vi "DFD Filter Array.vi"(7 "init (F)":bool, 8 "error in (no error)":errorcluster, 10 "filters":T1[](array[typedef]) {"mSRate_QSettings"."source" items=["Coef a/k"=0, "Coef b/v"=7, "Input"=1, "Output"=2, "Multiplicand"=3, "Product"=4, "Sum"=5, "Delay"=6, "Gain"=8]}, 11 "signal in":waveform(dbl)[](array[waveform])) -> (0 "error out":errorcluster, 3 "signal out":waveform(dbl)[](array[waveform]))   [LabVIEW 2019, in "Instrument.Lockin.lvlib" / "Instrument.DAQ.lvclass"]
uses:
  Instrument.DAQ.lvclass
  <vilib>/addons/Digital Filter Design/_Objects.llb/DFD Filter Obj.ctl
  <vilib>/addons/Digital Filter Design/_Objects.llb/DFD Filter Coef.ctl
  <vilib>/addons/Digital Filter Design/_Objects.llb/DFD Filter Structure Type Selector.ctl
  <vilib>/addons/Digital Filter Design/_Objects.llb/dfd_Internal Quantization Settings.ctl
  <vilib>/addons/Digital Filter Design/_Objects.llb/dfd_Internal Quantization Srcs.ctl
  <vilib>/addons/Digital Filter Design/_Objects.llb/DFD Coef Norm Type.ctl
  <vilib>/addons/Digital Filter Design/Process.llb/DFD Filtering with State (Wfm).vi
  <vilib>/addons/Digital Filter Design/NI_DigFilterLicensed.lvlib
  <vilib>/addons/Digital Filter Design/NI_DigFilter_Process.lvlib
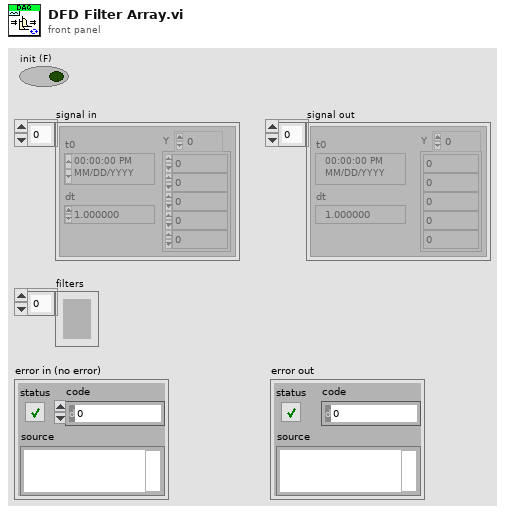
[diagram p1: front panel]
types:
  T1 = typedef "NI_DigFilterLicensed.lvlib/DFD Filter Obj.ctl" = cluster{"mSRate_Fs":dbl, "mSRate_Version":string, "mSRate_Comments":string, "mSRate_OrgCoef":T2, "mSRate_CurCoef":T2, "mSRate_Quantized?":bool, "mSRate_QCoef":T2, "mSRate_QSettings":T4[], "mSRate_Order":i32, "mSRate_Scaling":cluster{"mSRate_ScaleByPowerOf2?":bool, "mSRate_ScaleType":T6}}
  T2 = typedef "NI_DigFilterLicensed.lvlib/DFD Filter Coef.ctl" = cluster{"type":T3, "gain":dbl, "coef a (k)":dbl[], "coef b (v)":dbl[]}
  T3 = typedef "NI_DigFilterLicensed.lvlib/DFD Filter Structure Type Selector.ctl" = enum16{"Undefined", "FIR Direct Form", "FIR Direct Form Transposed", "FIR Symmetric", "FIR Antisymmetric", "IIR Direct Form I", "IIR Direct Form I Transposed", "IIR Direct Form II", "IIR Direct Form II Transposed", "IIR Cascaded Second Order Sections Form I", "IIR Cascaded Second Order Sections Form I Transposed", "IIR Cascaded Second Order Sections Form II", "IIR Cascaded Second Order Sections Form II Transposed", "Lattice Allpass (basic sections)", "Lattice Allpass (one multiplier sections)", "Lattice Allpass (normalized sections)", "Lattice AR (basic sections)", "Lattice AR (one multiplier sections)", "Lattice AR (normalized sections)", "Lattice MA (minimum phase)", "Lattice MA (maximum phase)", "Lattice ARMA (basic sections)", "Lattice ARMA (one multiplier sections)", "Lattice ARMA (normalized sections)"}
  T4 = typedef "NI_DigFilterLicensed.lvlib/dfd_Internal Quantization Settings.ctl" = cluster{"source":T5, "wl":i16, "iwl":i16, "overflow mode":enum16{"Saturation", "Wrap"}, "rounding mode":enum16{"Nearest", "Truncation"}, "signed?":bool}
  T5 = typedef "NI_DigFilterLicensed.lvlib/dfd_Internal Quantization Srcs.ctl" = u16
  T6 = typedef "NI_DigFilterLicensed.lvlib/DFD Coef Norm Type.ctl" = enum16{"No Norm", "Time Domain 1-Norm", "Time Domain 2-Norm", "Time Domain Inf-Norm"}
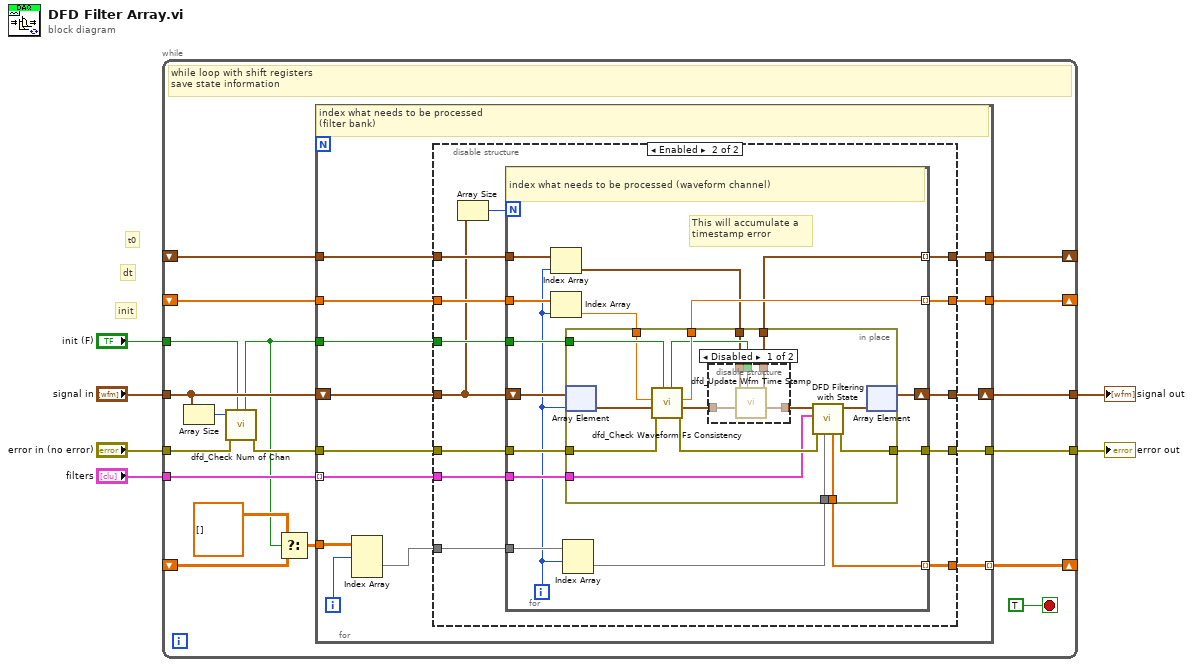
[diagram p0: block diagram]
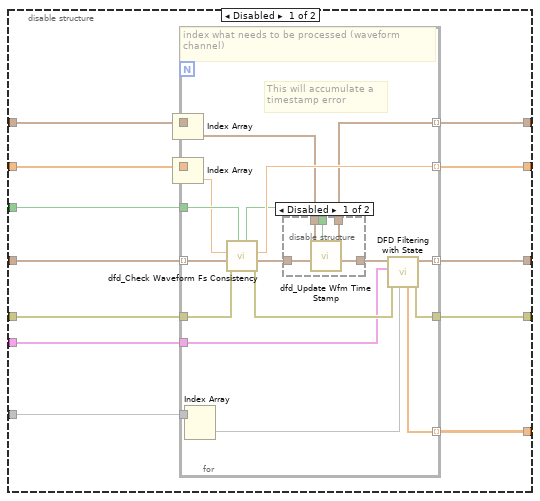
[diagram p2: hidden frame]
diagram:
  # "t0"
  # "dt"
  # "init"
  n1 = while {
    tunnel: "init (F)" -> [w10]
    tunnel: "filters" -> [w22]
    shift-right: [w20] -> _
    shift-left: _ -> [w19]
    tunnel: "error in (no error)" -> [w8]
    tunnel: [w23] -> w2
    tunnel: "signal in" -> [w11]
    tunnel: [w24] -> w1
    shift-right: [w15] -> _
    shift-left: _ -> [w13]
    shift-right: [w16] -> _
    shift-left: _ -> [w14]
    stop <- TRUE stop-if-true
    # "while loop with shift registers \nsave state information"
    n2 = Array Size(array=w11) -> (size(s)=w12:i32)
    n3 = call <vilib>:"dfd_Check Num of Chan.vi"("init in"=w10, "error in (no error)"=w8, "#ch in"=w12) -> ("error out"=w9:errorcluster, "init out"=w7:bool)  [unwired: 7 out]
    n4 = Select(t=dbl[][][] [], s=w7, f=w19) -> (s? t:f=w17:dbl[][][])
    n5 = for {
      tunnel: w22 -> [w34] mode=indexing
      tunnel: [w33] -> w20 mode=indexing
      tunnel: w9 -> [w36]
      tunnel: [w37] -> w23
      tunnel: w17 -> [w32]
      tunnel: w7 -> [w30]
      shift-right: [w38] -> w24
      shift-left: w11 -> [w35]
      tunnel: [w29] -> w16
      tunnel: [w28] -> w15
      tunnel: w14 -> [w27]
      tunnel: w13 -> [w26]
      i -> [w31]
      # "index what needs to be processed\n(filter bank)"
      n6 = Index Array(array=w32, index (dim 0)=w31) -> (element=w25:dbl[][])  [unwired: 2 in]
      n7 = disable-structure shown="Enabled" {
        disable-tunnel: [w50 w89] -> w38
        disable-tunnel: [w49 w88] -> w37
        disable-tunnel: w36 -> [w48 w87]
        disable-tunnel: w35 -> [w47 w78]
        disable-tunnel: w34 -> [w46 w86]
        disable-tunnel: [w45 w85] -> w33
        disable-tunnel: w30 -> [w44 w84]
        disable-tunnel: [w43 w83] -> w29
        disable-tunnel: [w42 w82] -> w28
        disable-tunnel: w27 -> [w41 w81]
        disable-tunnel: w26 -> [w40 w80]
        disable-tunnel: w25 -> [w39 w79]
        frame Disabled {
          n8 = for {
            tunnel: [w70] -> w45 mode=indexing
            tunnel: w39 -> [w69]
            tunnel: w46 -> [w58]
            tunnel: w48 -> [w65]
            tunnel: [w51] -> w49
            tunnel: w47 -> [w67] mode=indexing
            tunnel: [w55] -> w50 mode=indexing
            tunnel: w44 -> [w64]
            tunnel: [w63] -> w42 mode=indexing
            tunnel: [w54] -> w43 mode=indexing
            tunnel: w41 -> [w62]
            tunnel: w40 -> [w61]
            i -> [w59]
            # "This will accumulate a \ntimestamp error"
            # "index what needs to be processed (waveform channel)"
            n9 = Index Array(array=w62, index=w59) -> (element=w56:timestamp)
            n10 = Index Array(array=w61, index=w59) -> (element=w57:dbl)
            n11 = Index Array(array=w69, index (row)=w59) -> (element=w68:dbl[])  [unwired: 1 in]
            n12 = call <vilib>:"dfd_Check Waveform Fs Consistency.vi"("init in"=w64, "error in (no error)"=w65, "signal in"=w67, "dt in"=w57) -> ("error out"=w66:errorcluster, "signal out"=w53:waveform(dbl), "dt out"=w63:dbl, "init out"=w60:bool)  [unwired: 4 out]
            n13 = disable-structure shown="Disabled" {
              disable-tunnel: w60 -> [w75 _]
              disable-tunnel: w56 -> [w74 _]
              disable-tunnel: [w73 _] -> w54
              disable-tunnel: w53 -> [w72 w76]
              disable-tunnel: [w71 w76] -> w52
              frame Disabled {
                n14 = call <vilib>:"dfd_Update Wfm Time Stamp.vi"("init? (F)"=w75, "signal in"=w72, "t0"=w74) -> ("signal out"=w71:waveform(dbl), "tf"=w73:timestamp)  [unwired: 1 in, 6 out]
              }
              frame Enabled {
              }
            }
            n15 = call-poly <vilib>:"DFD Filtering with State.vi"("state in"=w68, "error in (no error)"=w66, "filter"=w58, "signal in"=w52) -> ("error out"=w51:errorcluster, "signal out"=w55:waveform(dbl), "state out"=w70:dbl[])  [unwired: 5 in]
          }
        }
        frame Enabled {
          n16 = Array Size(array=w78) -> (size(s)=w77:i32)
          n17 = for {
            N: w77 -> [_]
            tunnel: [w105] -> w85 mode=indexing
            tunnel: w79 -> [w104]
            tunnel: w86 -> [w97]
            tunnel: w87 -> [w102]
            tunnel: [w93] -> w88
            tunnel: w84 -> [w101]
            tunnel: [w100] -> w82 mode=indexing
            tunnel: [w94] -> w83 mode=indexing
            tunnel: w81 -> [w99]
            tunnel: w80 -> [w98]
            shift-right: [w91] -> w89
            shift-left: w78 -> [w92]
            i -> [w90]
            # "This will accumulate a \ntimestamp error"
            # "index what needs to be processed (waveform channel)"
            n18 = Index Array(array=w99, index=w90) -> (element=w95:timestamp)
            n19 = Index Array(array=w98, index=w90) -> (element=w96:dbl)
            n20 = Index Array(array=w104, index (row)=w90) -> (element=w103:dbl[])  [unwired: 1 in]
            n21 = in-place {
              in-place-border: [w121] -> w105
              in-place-border: w103 -> [w120]
              in-place-border: w102 -> [w118]
              in-place-border: w101 -> [w117]
              in-place-border: [w116] -> w100
              in-place-border: w97 -> [w114]
              in-place-border: w96 -> [w113]
              in-place-border: w95 -> [w112]
              in-place-border: [w111] -> w94
              in-place-border: [w108] -> w93
              n22 = in-place-array #1(w92, w90) -> (w107:waveform(dbl))
              n23 = call <vilib>:"dfd_Check Waveform Fs Consistency.vi"("init in"=w117, "error in (no error)"=w118, "signal in"=w107, "dt in"=w113) -> ("error out"=w119:errorcluster, "signal out"=w110:waveform(dbl), "dt out"=w116:dbl, "init out"=w115:bool)  [unwired: 4 out]
              n24 = disable-structure shown="Disabled" {
                disable-tunnel: w115 -> [w126 _]
                disable-tunnel: w112 -> [w125 _]
                disable-tunnel: [w124 _] -> w111
                disable-tunnel: w110 -> [w123 w127]
                disable-tunnel: [w122 w127] -> w109
                frame Disabled {
                  n25 = call <vilib>:"dfd_Update Wfm Time Stamp.vi"("init? (F)"=w126, "signal in"=w123, "t0"=w125) -> ("signal out"=w122:waveform(dbl), "tf"=w124:timestamp)  [unwired: 1 in, 6 out]
                }
                frame Enabled {
                }
              }
              n26 = call-poly <vilib>:"DFD Filtering with State.vi"("state in"=w120, "error in (no error)"=w119, "filter"=w114, "signal in"=w109) -> ("error out"=w108:errorcluster, "signal out"=w106:waveform(dbl), "state out"=w121:dbl[])  [unwired: 5 in]
              n27 = in-place-array #1(w106) -> (w91:waveform(dbl)[])  [unwired: 1 out]
            }
          }
        }
      }
    }
  }
  "error out" <- w2
  "signal out" <- w1
